vi "Edit Auton Queue Order.vi"(10 "Boolean":bool, 11 "Manip Button":T1) -> ()   [LabVIEW 2015]
uses:
  Common Code/Gamepads/Button Cluster.ctl
  Common Code/Change Detect Boolean.vi
  Robot Global Data.vi
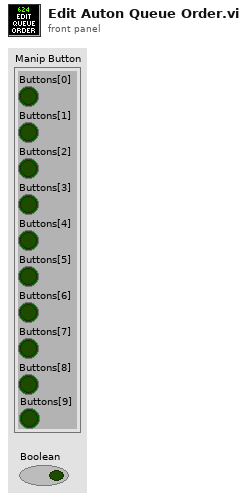
[diagram p1: front panel]
types:
  T1 = typedef "Button Cluster.ctl" = cluster{"Buttons[0]":bool, "Buttons[1]":bool, "Buttons[2]":bool, "Buttons[3]":bool, "Buttons[4]":bool, "Buttons[5]":bool, "Buttons[6]":bool, "Buttons[7]":bool, "Buttons[8]":bool, "Buttons[9]":bool}
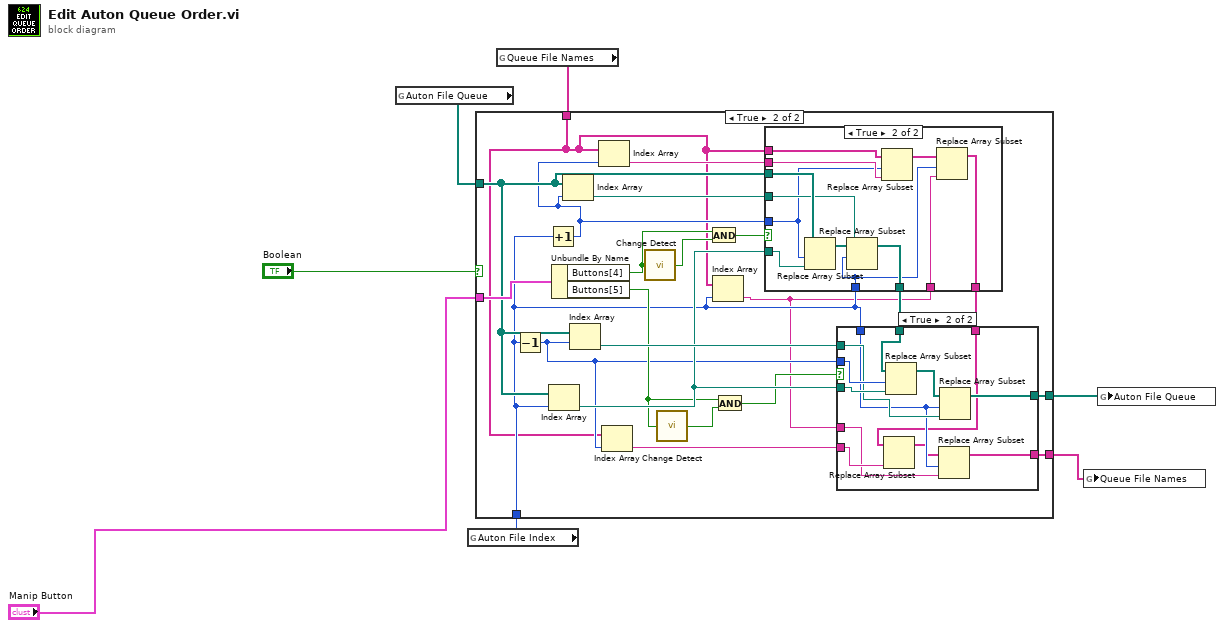
[diagram p0: block diagram]
diagram:
  n1 = global read "Robot Global Data.vi" "Auton File Queue"() -> (w6:path[])
  n2 = global read "Robot Global Data.vi" "Auton File Index"() -> (w5:i32)
  n3 = global read "Robot Global Data.vi" "Queue File Names"() -> (w2:string[])
  n4 = case shown="True" "Boolean" {
    tunnel: "Manip Button" -> [_ w31]
    tunnel: w5 -> [_ w14]
    tunnel: w6 -> [w9 w30]
    tunnel: [w9 w25] -> w7
    tunnel: w2 -> [w8 w13]
    tunnel: [w8 w10] -> w1
    frame False {
    }
    frame True {
      n5 = Decrement(x=w14) -> (x-1=w17:i32)
      n6 = Increment(x=w14) -> (x+1=w18:i32)
      n7 = Index Array(array=w30, index=w14) -> (element=w27:path)
      n8 = Unbundle By Name(w31) -> ("Buttons[4]"=w23:bool, "Buttons[5]"=w21:bool)
      n9 = Index Array(array=w30, index=w18) -> (element=w29:path)
      n10 = Index Array(array=w30, index=w17) -> (element=w28:path)
      n11 = Index Array(array=w13, index=w18) -> (element=w15:string)
      n12 = Index Array(array=w13, index=w17) -> (element=w16:string)
      n13 = call-poly "Change Detect.vi"("In"=w23) -> ("Changed?"=w24:bool)
      n14 = call-poly "Change Detect.vi"("In"=w21) -> ("Changed?"=w20:bool)
      n15 = And(x=w23, y=w24) -> (x .and. y?=w22:bool)
      n16 = Index Array(array=w13, index=w14) -> (element=w11:string)
      n17 = And(x=w21, y=w20) -> (x .and. y?=w19:bool)
      n18 = case shown="True" w22 {
        tunnel: w30 -> [w47 w59]
        tunnel: w18 -> [_ w49]
        tunnel: w27 -> [_ w58]
        tunnel: w29 -> [_ w56]
        tunnel: w14 -> [_ w48]
        tunnel: [w47 w55] -> w26
        tunnel: w15 -> [_ w53]
        tunnel: w13 -> [w46 w54]
        tunnel: w11 -> [_ w51]
        tunnel: [w46 w50] -> w12
        frame False {
        }
        frame True {
          n19 = Replace Array Subset(array=w59, new element=w58, index=w49) -> (w57:path[])
          n20 = Replace Array Subset(array=w57, new element=w56, index=w48) -> (w55:path[])
          n21 = Replace Array Subset(array=w54, new element=w53, index=w49) -> (w52:string[])
          n22 = Replace Array Subset(array=w52, new element=w51, index=w48) -> (w50:string[])
        }
      }
      n23 = case shown="True" w19 {
        tunnel: w14 -> [_ w39]
        tunnel: w28 -> [_ w41]
        tunnel: w27 -> [_ w44]
        tunnel: w26 -> [w33 w45]
        tunnel: w17 -> [_ w43]
        tunnel: [w33 w40] -> w25
        tunnel: w16 -> [_ w36]
        tunnel: w12 -> [w32 w38]
        tunnel: w11 -> [_ w35]
        tunnel: [w32 w34] -> w10
        frame False {
        }
        frame True {
          n24 = Replace Array Subset(array=w38, new element=w36) -> (w37:string[])  [unwired: 1 in]
          n25 = Replace Array Subset(array=w45, new element=w44, index=w43) -> (w42:path[])
          n26 = Replace Array Subset(array=w37, new element=w35, index=w39) -> (w34:string[])
          n27 = Replace Array Subset(array=w42, new element=w41, index=w39) -> (w40:path[])
        }
      }
    }
  }
  n28 = global write "Robot Global Data.vi" "Queue File Names"(w1) -> ()
  n29 = global write "Robot Global Data.vi" "Auton File Queue"(w7) -> ()
